vi "Read Configuration Parameters.vi"(8 "error in (no error)":errorcluster, 10 "refnum":T1, 11 "Example Configuration Dialog in":refnum<class "LogicIO Configuration.lvclass">) -> (0 "error out":errorcluster, 2 "refnum out":T1, 3 "Example Configuration Dialog out":refnum<class "LogicIO Configuration.lvclass">)   [LabVIEW 2016, in "Hardware.lvlib" / "LogicIO.lvlib" / "LogicIO Configuration.lvclass"]
uses:
  <userlib>/Common Components/Hardware/LogicIO/LogicIO Config/LogicIO Configuration.lvclass
  <vilib>/Utility/config.llb/Config Data RefNum.ctl
  <userlib>/Common Components/Hardware/LogicIO/LogicIO Config/LogicIO Configuration.lvclass/LogicIO Configuration.ctl
  <userlib>/Common Components/Hardware/Abstract Hardware/Hardware.lvclass/Hardware.ctl
  <userlib>/Common Components/Hardware/Abstract Hardware/Read Label.vi
  <userlib>/Common Components/Hardware/LogicIO/LogicIO/LogicIO.lvclass
  C:/Program Files (x86)/National Instruments/LabVIEW 2016/user.lib/Common Components/Hardware/Abstract Hardware/Hardware.lvclass
  <vilib>/Utility/config.llb/NI_LVConfig.lvlib
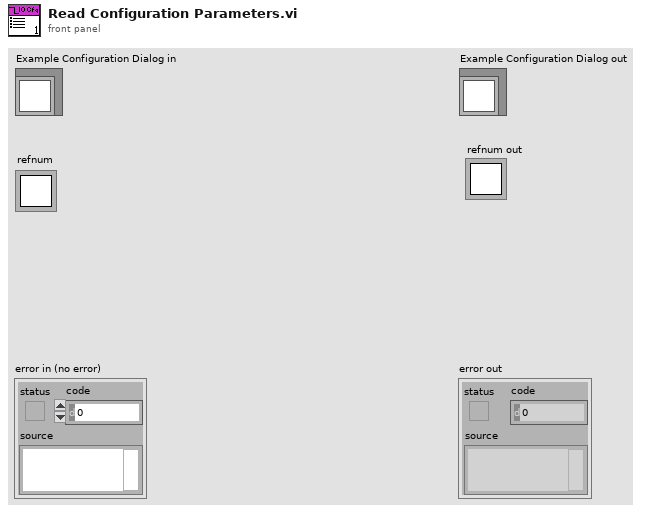
[diagram p1: front panel]
types:
  T1 = typedef "NI_LVConfig.lvlib/Config Data RefNum.ctl" = refnum<k1>
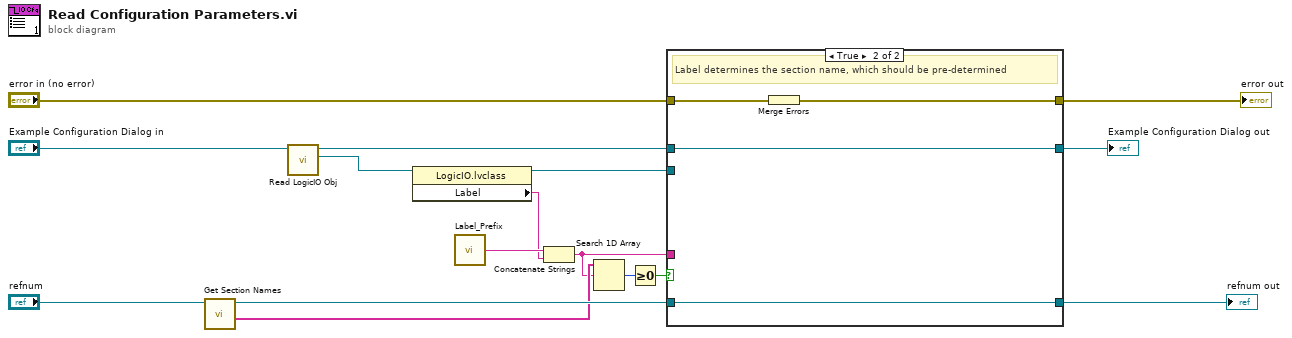
[diagram p0: block diagram]
diagram:
  n1 = call <vilib>:"Get Section Names.vi"("refnum"="refnum") -> ("section names"=w6:string[], "refnum out"=w7:T1)  [unwired: 8 in, 1 out]
  n2 = call <userlib>:"Read LogicIO Obj.vi"("LogicIO Configuration in"="Example Configuration Dialog in") -> ("Hardware.lvlib:LogicIO.lvlib:LogicIO.lvclass"=w8:refnum<class "LogicIO.lvclass">, "LogicIO Configuration out"=w10:refnum<class "LogicIO Configuration.lvclass">)  [unwired: 9 in]
  n3 = property class="LogicIO.lvclass"(reference=w8) -> (reference out=w1:refnum<class "LogicIO.lvclass">, "Label"=w2:string)  [unwired: 1 in, 1 out]
  n4 = call <userlib>:"Label_Prefix.vi"() -> ("Label Prefix String"=w9:string)
  n5 = Concatenate Strings(w9, w2) -> (w5:string)
  n6 = Search 1D Array(1D array=w6, element=w5) -> (index of element=w4:i32)  [unwired: 1 in]
  n7 = Greater Or Equal To 0?(x=w4) -> (x >= 0?=w3:bool)
  n8 = case shown="True" w3 {
    tunnel: w7 -> [w18 w23]
    tunnel: "error in (no error)" -> [w17 w20]
    tunnel: w10 -> [w19 w21]
    tunnel: [w19 w21] -> w14
    tunnel: [w18 w23] -> w13
    tunnel: [w17 w22] -> w12
    tunnel: w5 -> [_ _]
    tunnel: w1 -> [_ _]
    frame False {
    }
    frame True {
      # "Label determines the section name, which should be pre-determined"
      n9 = Merge Errors(w20) -> (w22:errorcluster)
    }
  }
  "Example Configuration Dialog out" <- w14
  "error out" <- w12
  "refnum out" <- w13
